vi "TestCloneAPI.vi"() -> ()   [LabVIEW 2014, in "PmuImpairModule.lvlib"]
uses:
  PmuImpairModule.lvlib
  PmuImpairPlugins/PmuImpairPluginBase_class/TypeDefs/clImpairConfig.ctl
  PublicAPI/Arguments/Requests/dblImpairParams.ctl
  EventPlugins/EventPluginBaseClass/TypeDefs/clEvtReportArray.ctl
  EventPlugins/EventPluginBaseClass/TypeDefs/clEvtReport.ctl
  EventPlugins/EventPluginBaseClass/TypeDefs/dblEvtSignalArray.ctl
  EventPlugins/EventPluginBaseClass/TypeDefs/clEvtConfig.ctl
  <userlib>/NIST/ModuleAdminLib/ModuleAdmin/ModuleAdmin.lvclass
  PublicAPI/Arguments/Broadcasts/clDidInit.ctl
  <userlib>/NIST/ModuleAdminLib/ModuleAdmin/ModuleAdmin.lvclass/ModuleAdmin.ctl
  PublicAPI/Arguments/Requests/clStopArgument.ctl
  PublicAPI/Arguments/Broadcasts/clStatUpdate.ctl
  PublicAPI/Arguments/Broadcasts/clErrorRpt.ctl
  <userlib>/NIST/ModuleAdminLib/ModuleAdmin/Accessors/Read CloneRegRef.vi
  <userlib>/NIST/ModuleAdminLib/CloneRegistration/CloneRegistration.lvclass
  PmuImpairPlugins/PmuImpairPluginBase_class/PmuImpairPluginBase.lvclass
  EventPlugins/EventPluginBaseClass/EventPluginBaseClass.lvclass
panel:
  in  "Show Panel":bool=TRUE
  in  "btnWriteEvtParams":bool caption="Write Impair Config"
  in  "dblEvtParams":dbl[][](array[numeric])=[[70.0, 20.0], [60.0, 60.0], [0.0, 0.0], [0.0, 0.0], [0.0, 0.0], [0.0, 0.0], [0.0, 0.0], [0.0, 0.0], [0.0, 0.0], [0.0, 0.0], [0.0, 0.0], [0.0, 0.0], [0.0, 0.0]]
  in  "btnWriteEventConfig":bool caption="Write Impair Config"
  in  "clEvtConfig":T1={"T0(UTC)"=0.0, "F0"=60.0, "Fs"=60, "FSamp"=960, "bPosSeq"=FALSE}
  in  "dblEventSignalArray":T2=[[98.99494936611666, 91.45940754134637, 70.00000000000001, 37.8837270102338, 2.80427866210764e-14, -37.88372701023376, -70.0, -91.45940754134637, -98.99494936611666, -91.45940754134638, -70.00000000000004, -37.88372701023385, -1.8184476598510646e-14, 37.883727010233734, 69.99999999999999, 91.45940754134634, 98.99494936611666, 91.4594075413464, 70.00000000000009, 37.88372701023394, 1.1823263868380915e-13, -37.883727010233635, -69.99999999999991, -91.45940754134627, -98.99494936611666, -91.45940754134637, -70.0000000000001, -37.88372701023387, -4.2430445396524844e-14, 37.88372701023363, 69.99999999999991, 91.45940754134627, 98.99494936611666, 91.45940754134637, 70.0000000000001, 37.883727010233876, 2.3040378516811477e-13, -37.88372701023378, -69.99999999999977, -91.45940754134632, -98.99494936611666, -91.45940754134644, -70.00000000000024, -37.88372701023389, -2.4252676956712185e-13, 37.88372701023344, 69.99999999999964, 91.45940754134625, 98.99494936611666, 91.45940754134644, 70.0, 37.8837270102339, 2.546497539661289e-13, -37.883727010233436, -69.99999999999989, -91.45940754134625, -98.99494936611666, -91.45940754134645, -70.00000000000026, -37.88372701023424, -2.6677273836513605e-13, 37.88372701023342, 69.99999999999962, 91.45940754134624, 98.99494936611666, 91.45940754134658, 70.00000000000001, 37.883727010233926, 2.7889572276414313e-13, -37.883727010233414, -69.99999999999986, -91.45940754134624, -98.99494936611666, -91.4594075413466, -70.00000000000001, -37.88372701023393, -6.427194179083158e-13, 37.88372701023307, 69.99999999999986, 91.45940754134622, 98.99494936611666, 91.45940754134645, 70.00000000000028, 37.88372701023427, 6.548424023073229e-13, -37.88372701023371, -69.99999999999986, -91.45940754134622, -98.99494936611666, -91.45940754134632, -70.00000000000054, -37.88372701023461, -1.0186660974514956e-12, 37.88372701023337, 69.99999999999959, 91.45940754134608, 98.99494936611666, 91.45940754134647, 70.0000000000003, 37.883727010234296, -2.431305038499409e-14, -37.883727010233684, -69.99999999999983, -91.45940754134621, -98.99494936611666, -91.45940754134661, -70.00000000000054, -37.88372701023463, -3.3951064475917863e-13, 37.88372701023335, 69.99999999999957, 91.45940754134607, 98.99494936611666, 91.45940754134648, 70.00000000000031, 37.88372701023432, 7.033343399033513e-13, -37.88372701023302, -69.99999999999932, -91.45940754134621, -98.99494936611666, -91.45940754134661, -70.00000000000057, -37.88372701023465, -1.0671580350475241e-12, 37.88372701023333, 69.99999999999956, 91.45940754134607, 98.99494936611666, 91.45940754134675, 70.00000000000082, 37.88372701023499, 2.41788872110343e-14, -37.88372701023364, -69.9999999999998, -91.4594075413462, -98.99494936611666, -91.45940754134662, -70.0000000000006, -37.88372701023468, -3.8800258235520704e-13, 37.88372701023331, 69.99999999999953, 91.45940754134607, 98.99494936611666, 91.45940754134676, 70.00000000000084, 37.88372701023371, 4.8424856009048493e-14, -37.88372701023362, -69.99999999999977, -91.45940754134593, -98.99494936611666, -91.4594075413469, -70.0000000000011, -37.88372701023405, -4.122485511532212e-13, 37.88372701023329, 69.99999999999952, 91.45940754134605, 98.99494936611666, 91.45940754134678, 70.00000000000036, 37.88372701023439, 7.760722462973939e-13, -37.88372701023295, -69.99999999999926, -91.45940754134591, -98.99494936611666, -91.4594075413469, -70.00000000000011, -37.88372701023407, -4.364945199512354e-13, 37.883727010233265, 69.9999999999995, 91.45940754134604, 98.99494936611666, 91.45940754134625, 69.99999999999989, 37.883727010233756, 1.5037196365857394e-12, -37.88372701023228, -69.99999999999875, -91.45940754134563, -98.99494936611666, -91.45940754134665, -70.00000000000064, -37.88372701023474, -1.1641419102395808e-12, 37.88372701023259, 69.99999999999899, 91.45940754134577, 98.99494936611666], [28.284271247461902, 26.13125929752753, 20.000000000000004, 10.823922002923942, 8.012224748878971e-15, -10.823922002923933, -20.0, -26.13125929752753, -28.284271247461902, -26.13125929752754, -20.00000000000001, -10.823922002923956, -5.1955647424316135e-15, 10.823922002923924, 19.999999999999996, 26.131259297527524, 28.284271247461902, 26.131259297527542, 20.000000000000025, 10.823922002923982, 3.3780753909659755e-14, -10.823922002923897, -19.99999999999998, -26.131259297527503, -28.284271247461902, -26.13125929752753, -20.00000000000003, -10.823922002923963, -1.2122984399007097e-14, 10.823922002923894, 19.999999999999975, 26.131259297527503, 28.284271247461902, 26.13125929752753, 20.000000000000032, 10.823922002923965, 6.582965290517564e-14, -10.823922002923938, -19.999999999999936, -26.13125929752752, -28.284271247461902, -26.131259297527553, -20.000000000000068, -10.823922002923968, -6.929336273346338e-14, 10.823922002923842, 19.999999999999897, 26.1312592975275, 28.284271247461902, 26.131259297527553, 20.0, 10.823922002923972, 7.275707256175113e-14, -10.823922002923839, -19.999999999999968, -26.1312592975275, -28.284271247461902, -26.131259297527556, -20.00000000000007, -10.823922002924068, -7.622078239003887e-14, 10.823922002923835, 19.999999999999893, 26.131259297527496, 28.284271247461902, 26.131259297527595, 20.000000000000004, 10.823922002923979, 7.968449221832661e-14, -10.823922002923831, -19.99999999999996, -26.131259297527496, -28.284271247461902, -26.131259297527595, -20.000000000000004, -10.82392200292398, -1.8363411940237595e-13, 10.823922002923736, 19.999999999999957, 26.131259297527492, 28.284271247461902, 26.13125929752756, 20.00000000000008, 10.823922002924077, 1.870978292306637e-13, -10.823922002923918, -19.999999999999957, -26.131259297527492, -28.284271247461902, -26.13125929752752, -20.000000000000153, -10.823922002924174, -2.9104745641471305e-13, 10.82392200292382, 19.999999999999883, 26.131259297527453, 28.284271247461902, 26.131259297527563, 20.000000000000085, 10.823922002924085, -6.9465858242840266e-15, -10.823922002923911, -19.99999999999995, -26.13125929752749, -28.284271247461902, -26.131259297527603, -20.000000000000156, -10.823922002924181, -9.700304135976532e-14, 10.823922002923815, 19.99999999999988, 26.13125929752745, 28.284271247461902, 26.131259297527567, 20.00000000000009, 10.82392200292409, 2.0095266854381467e-13, -10.82392200292372, -19.999999999999805, -26.131259297527485, -28.284271247461902, -26.131259297527603, -20.000000000000163, -10.823922002924187, -3.04902295727864e-13, 10.823922002923808, 19.999999999999872, 26.13125929752745, 28.284271247461902, 26.131259297527645, 20.000000000000234, 10.823922002924283, 6.908253488866942e-15, -10.823922002923897, -19.999999999999943, -26.131259297527485, -28.284271247461902, -26.131259297527606, -20.000000000000167, -10.823922002924194, -1.108578806729163e-13, 10.823922002923803, 19.99999999999987, 26.131259297527446, 28.284271247461902, 26.13125929752765, 20.00000000000024, 10.823922002923918, 1.3835673145442426e-14, -10.823922002923892, -19.999999999999936, -26.131259297527407, -28.284271247461902, -26.131259297527688, -20.000000000000313, -10.823922002924014, -1.1778530032949179e-13, 10.823922002923796, 19.999999999999865, 26.131259297527443, 28.284271247461902, 26.13125929752765, 20.000000000000103, 10.82392200292411, 2.2173492751354114e-13, -10.8239220029237, -19.999999999999787, -26.131259297527404, -28.284271247461902, -26.131259297527688, -20.000000000000032, -10.82392200292402, -1.2471271998606725e-13, 10.823922002923789, 19.999999999999858, 26.13125929752744, 28.284271247461902, 26.1312592975275, 19.999999999999968, 10.823922002923931, 4.2963418188163984e-13, -10.823922002923508, -19.999999999999645, -26.131259297527325, -28.284271247461902, -26.131259297527617, -20.00000000000018, -10.823922002924212, -3.32611974354166e-13, 10.823922002923599, 19.999999999999712, 26.13125929752736, 28.284271247461902]]
  in  "btnWriteEvtSignal":bool caption="Write Impair Config"
  in  "btnReadPathToPlugin":bool caption="Write Impair Config"
  out "PathToPluginIniFileReport":path=path "P:/Framework/PmuImpairment/PmuImpairPlugins/SineModelPlugin/SineModelPlugin.ini"
  in  "btnGetImpairReports":bool caption="Write Impair Config"
  out "ImpairReportArray":T3 {"Synx" format="%#_4g"}
  in  "btnWriteEvtReports":bool caption="Write Impair Config"
  in  "EvtReportArray":T3=[{"Timestamp"=0.0, "Synx"=[70.0+0.0i, 35.0-60.6218i, 35.0+60.6218i], "Freq"=59.9, "ROCOF"=0.0, "ID"=0}, {"Timestamp"=0.02, "Synx"=[69.9962-0.733i, 34.3633-60.985i, 35.6329+60.2519i], "Freq"=59.9, "ROCOF"=0.0, "ID"=0}, {"Timestamp"=0.03, "Synx"=[69.9846-1.466i, 33.7228-61.3415i, 36.2619+59.8755i], "Freq"=59.9, "ROCOF"=0.0, "ID"=0}, {"Timestamp"=0.05, "Synx"=[69.9655-2.1988i, 33.0786-61.6912i, 36.8869+59.4925i], "Freq"=59.9, "ROCOF"=0.0, "ID"=0}] {"Synx" format="%#_4g"}
  in  "btnReadImpairParams":bool caption="Write Impair Config"
  out "dblImpairParamsReport":T5
  in  "btnWriteImpairParams":bool caption="Write Impair Config"
  in  "dblImpairParams":T5=[[8.19], [164.0]]
  in  "btnReadImpairConfig":bool caption="Write Impair Config"
  out "clImpairConfigReport":T6={"FilterType"="", "bPosSeq"=TRUE}
  in  "btnWriteImpairConfig":bool caption="Write Impair Config"
  in  "btnLoadPlugin":bool
  in  "PathToPluginIniFile":path=path "D:/Projects/PARTF/Framework/PmuImpairment/PmuImpairPlugins/C37BehaviourPlugin/C37BehaviourPlugin.ini"
  in  "clImpairConfig":T6={"FilterType"="Hamming", "bPosSeq"=TRUE}
  in  "btnRemove":bool
  out "Status Log":string
  out "Active Modules (Array)":string[](array[string])
  in  "btnAdd":bool
  in  "btnStop":bool
  in  "Select Module":i32(ring)=-1 caption="Select Module to send Request" items=["All"=-1]
  # "Hidden"
  # "Visible"
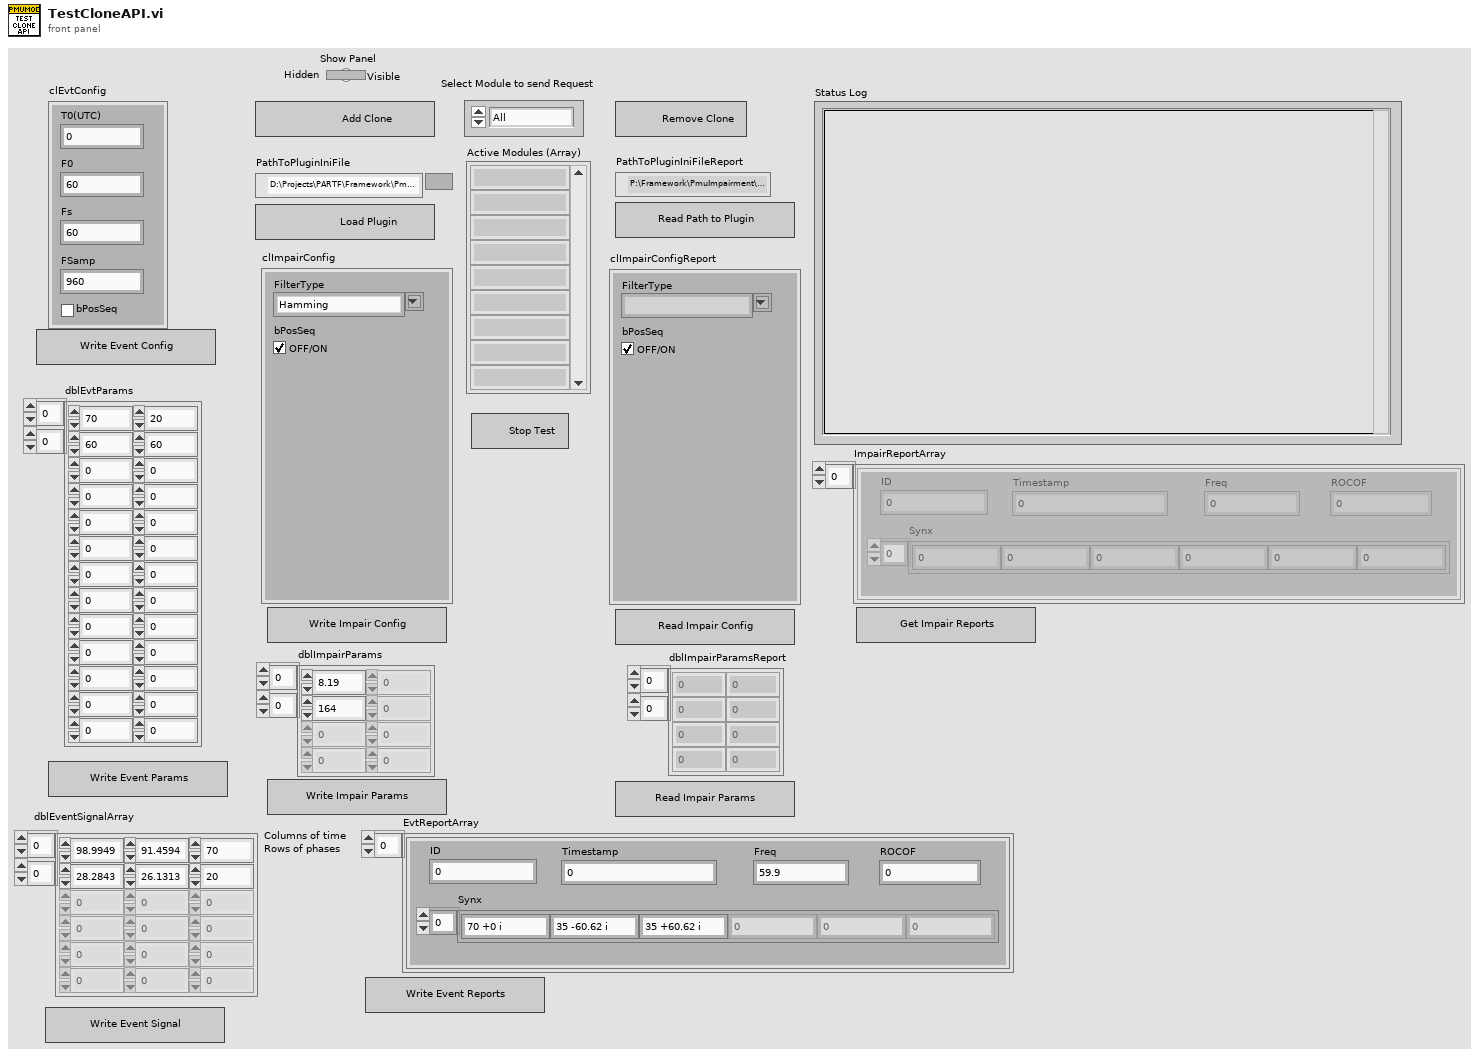
[diagram p1: front panel]
types:
  T1 = typedef "EventPlugins.lvlib/EventPluginBaseClass.lvclass/clEvtConfig.ctl" = cluster{"T0(UTC)":dbl, "F0":dbl, "Fs":i32, "FSamp":u32, "bPosSeq":bool}
  T2 = typedef "EventPlugins.lvlib/EventPluginBaseClass.lvclass/dblEvtSignalArray.ctl" = dbl[][]
  T3 = typedef "EventPlugins.lvlib/EventPluginBaseClass.lvclass/clEvtReportArray.ctl" = T4[]
  T4 = typedef "EventPlugins.lvlib/EventPluginBaseClass.lvclass/clEvtReport.ctl" = cluster{"Timestamp":dbl, "Synx":cdb[], "Freq":dbl, "ROCOF":dbl, "ID":i16}
  T5 = typedef "PmuImpairModule.lvlib/dblImpairParams.ctl" = dbl[][]
  T6 = typedef "PmuImpairPlugins.lvlib/PmuImpairPluginBase.lvclass/clImpairConfig.ctl" = cluster{"FilterType":string, "bPosSeq":bool}
  T7 = typedef "PmuImpairModule.lvlib/clBroadcastEvents.ctl" = cluster{"DidInit":refnum<user-event>, "StatusUpdate":refnum<user-event>, "ErrorReport":refnum<user-event>, "DidStop":refnum<user-event>, "ImpairConfig":refnum<user-event>, "ImpairParams":refnum<user-event>, "ImpairReports":refnum<user-event>, "PathToPlugin":refnum<user-event>, "BusNumber":refnum<user-event>}
  T8 = typedef "PmuImpairModule.lvlib/clDidInit.ctl" = cluster{"Init?":bool, "ModuleAdmin":refnum<class "ModuleAdmin.lvclass">}
  T9 = typedef "PmuImpairModule.lvlib/clStopArgument.ctl" = cluster{"Exit via Stop Module Req?":bool, "Wait for Module to stop?":bool, "ModuleAdmin":refnum<class "ModuleAdmin.lvclass">}
  T10 = typedef "PmuImpairModule.lvlib/clStatUpdate.ctl" = cluster{"Status":string}
  T11 = typedef "PmuImpairModule.lvlib/clErrorRpt.ctl" = cluster{"error":errorcluster, "AdditionalInfo":string}
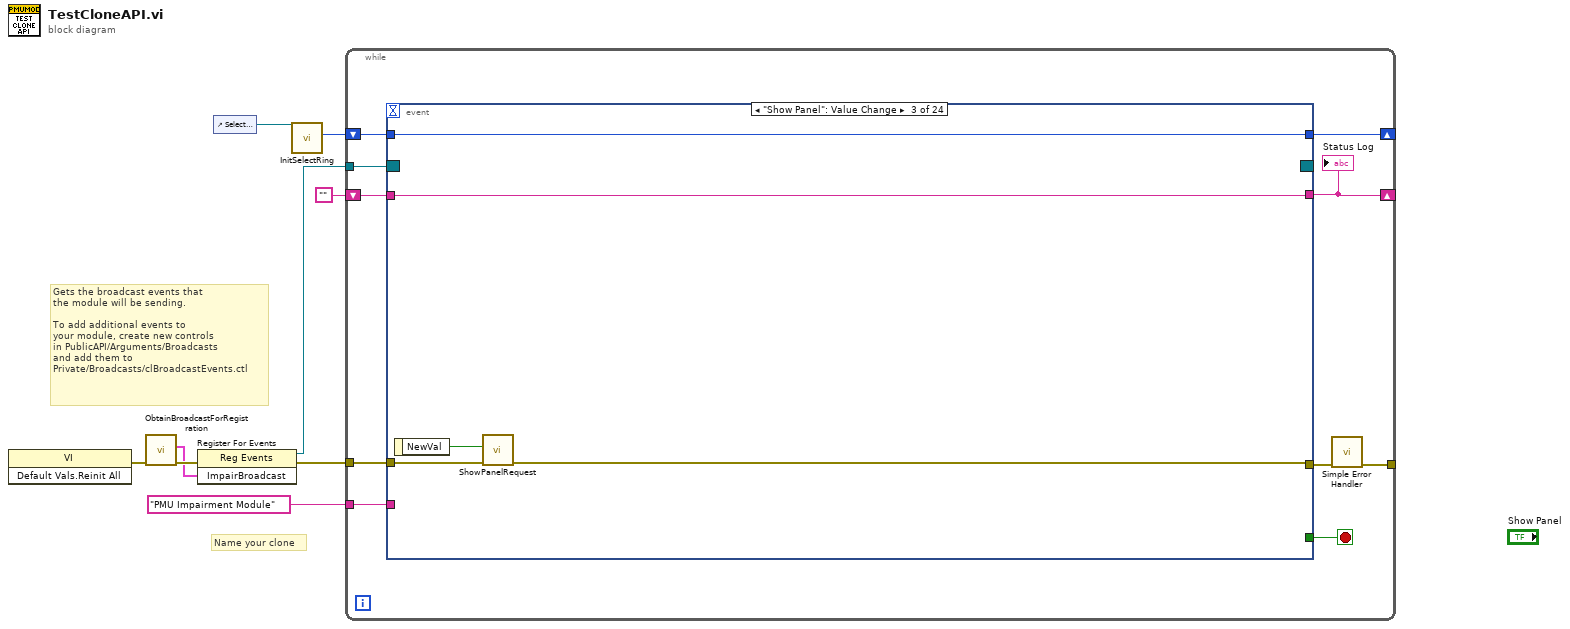
[diagram p0: block diagram]
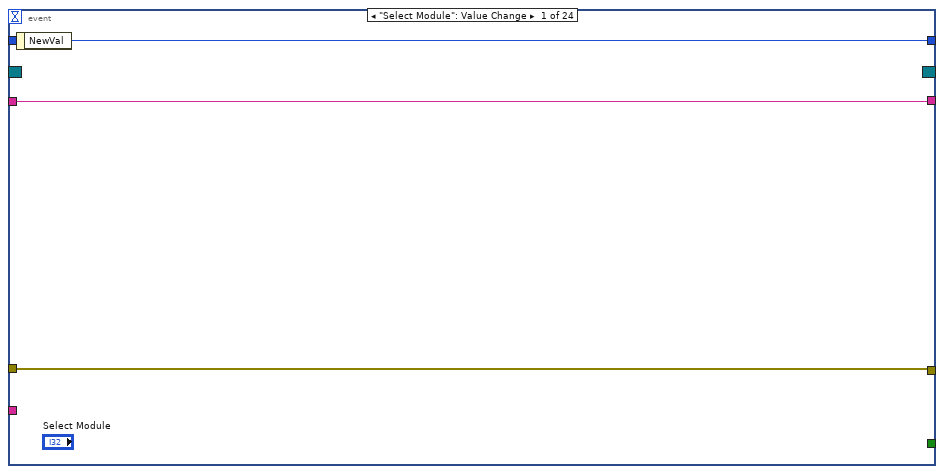
[diagram p2: hidden frame]
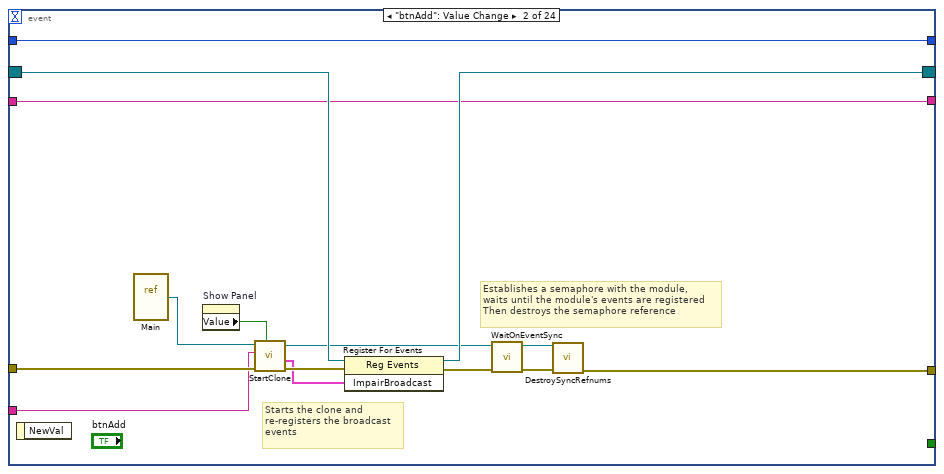
[diagram p3: hidden frame]
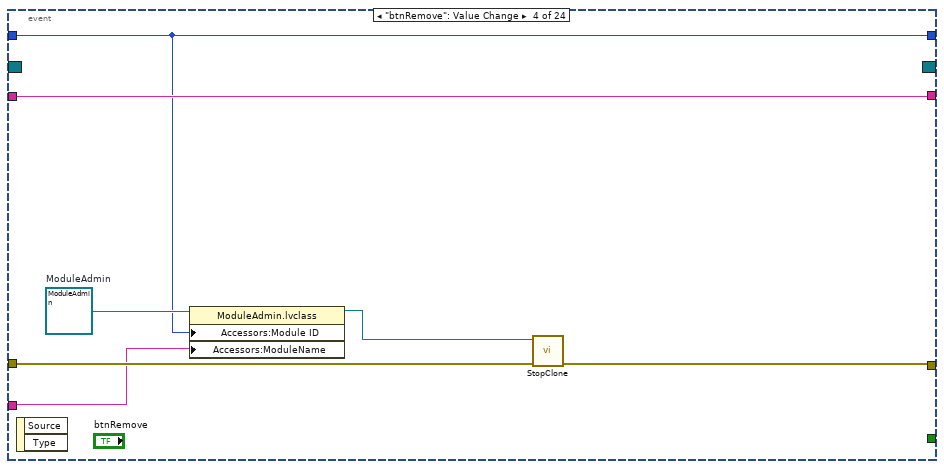
[diagram p4: hidden frame]
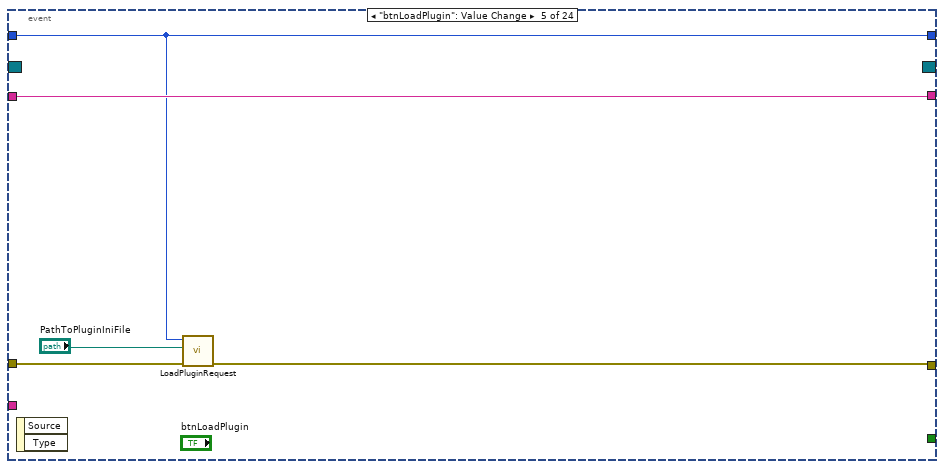
[diagram p5: hidden frame]
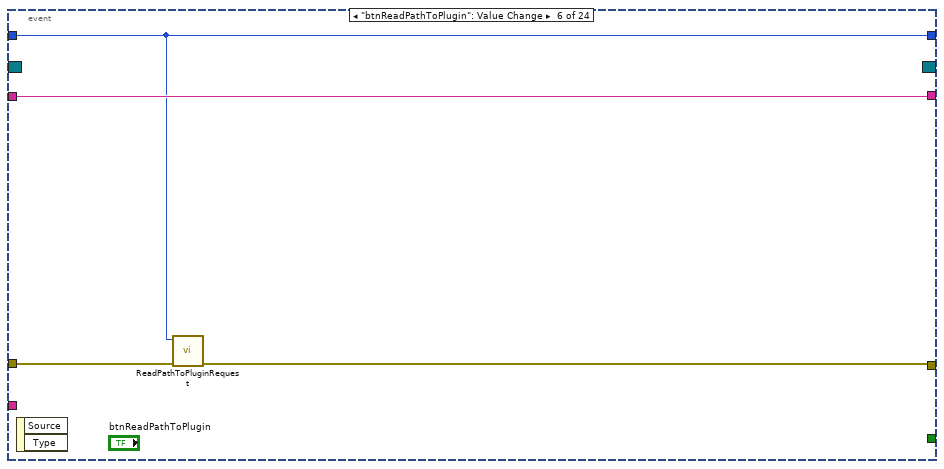
[diagram p6: hidden frame]
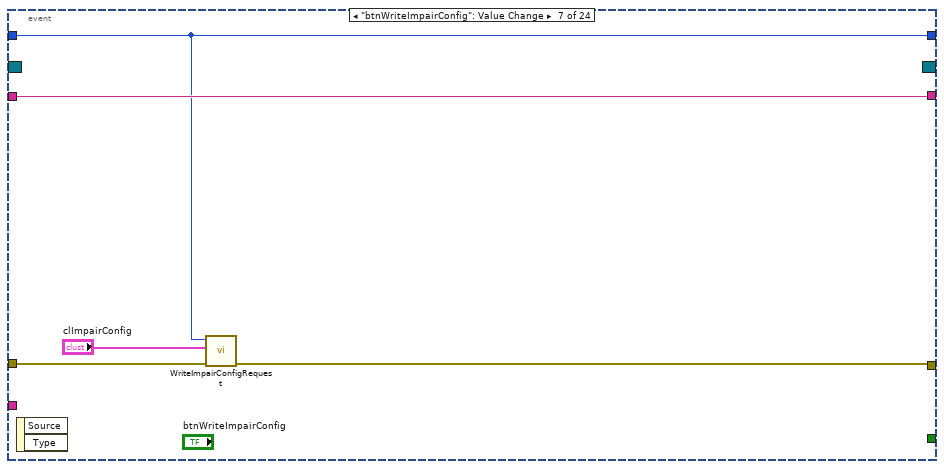
[diagram p7: hidden frame]
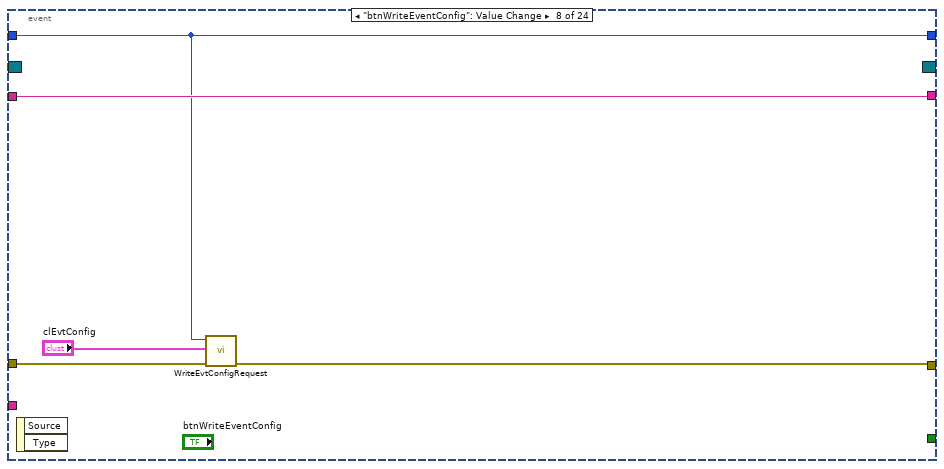
[diagram p8: hidden frame]
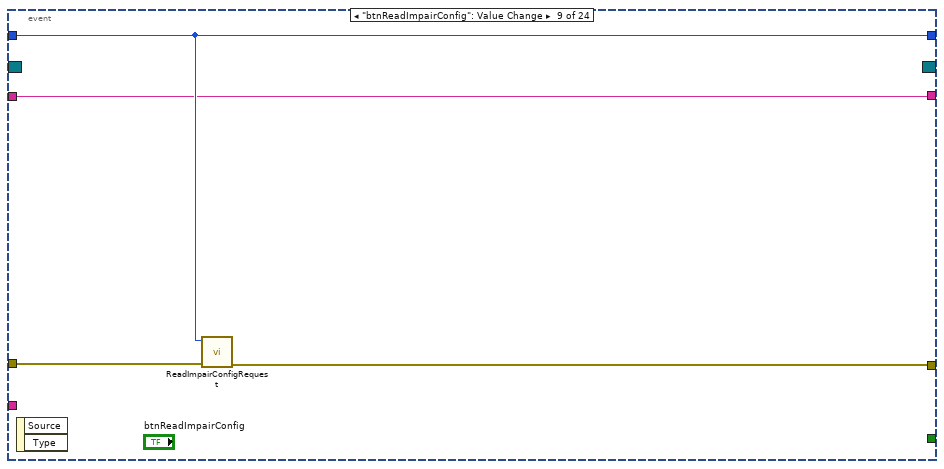
[diagram p9: hidden frame]
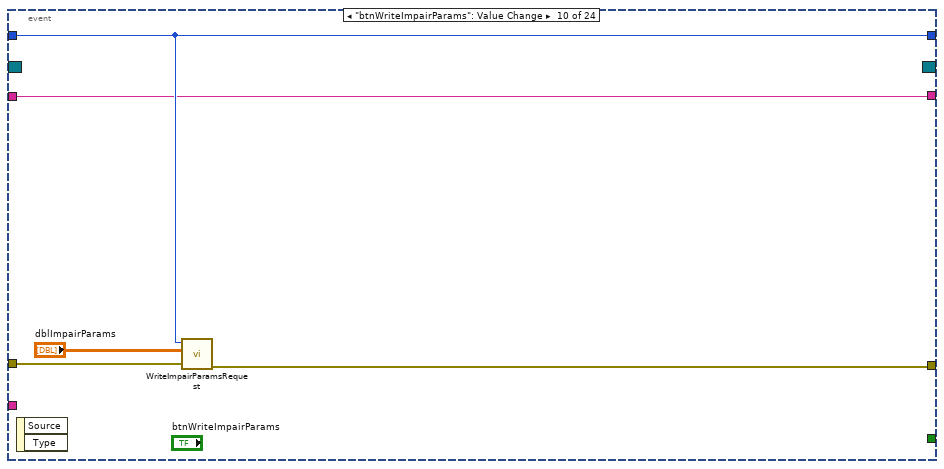
[diagram p10: hidden frame]
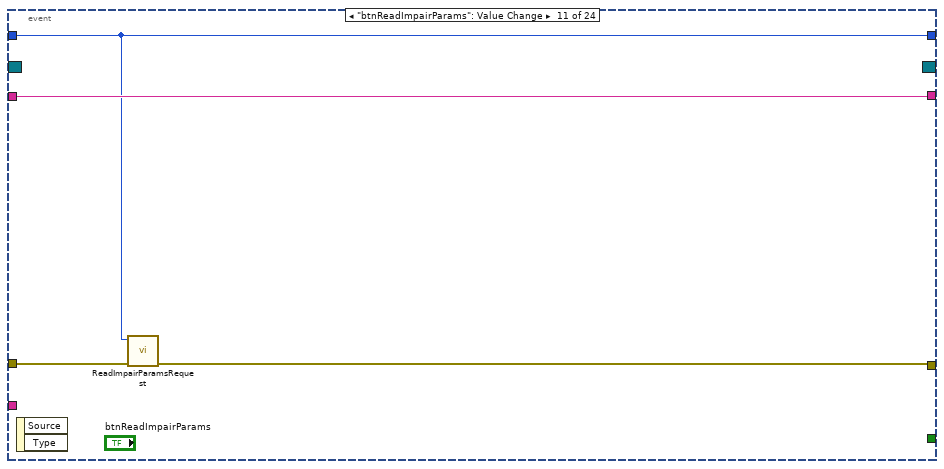
[diagram p11: hidden frame]
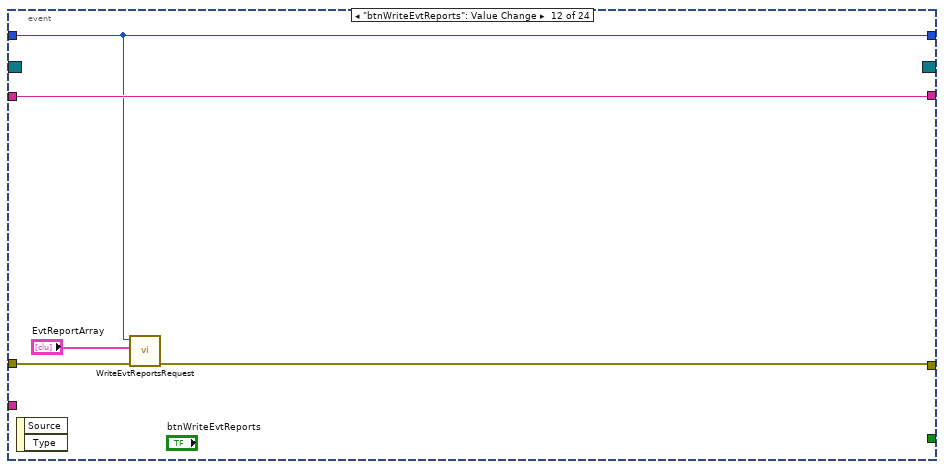
[diagram p12: hidden frame]
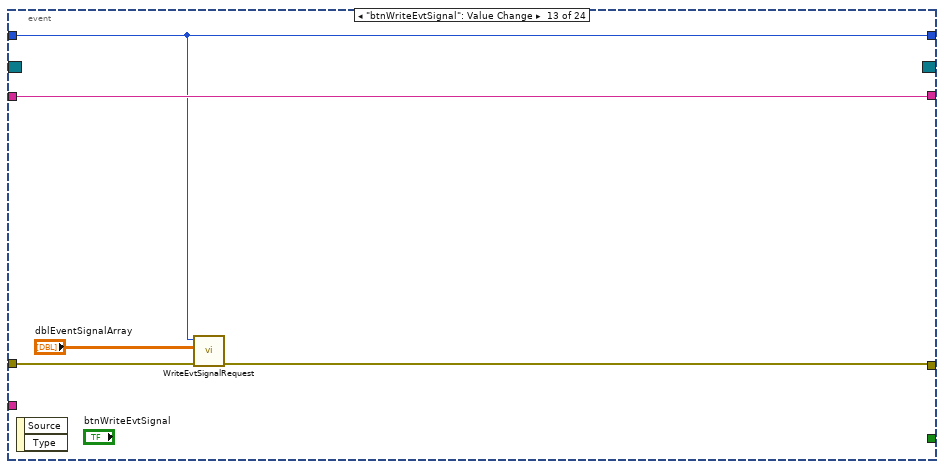
[diagram p13: hidden frame]
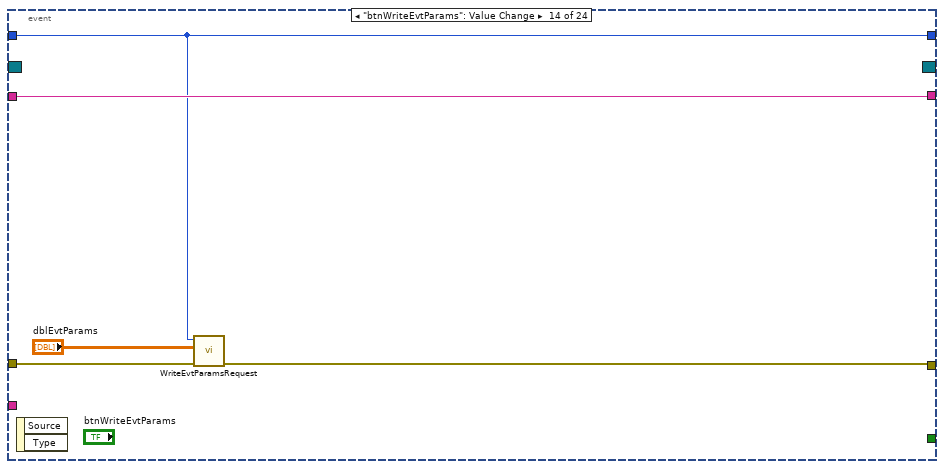
[diagram p14: hidden frame]
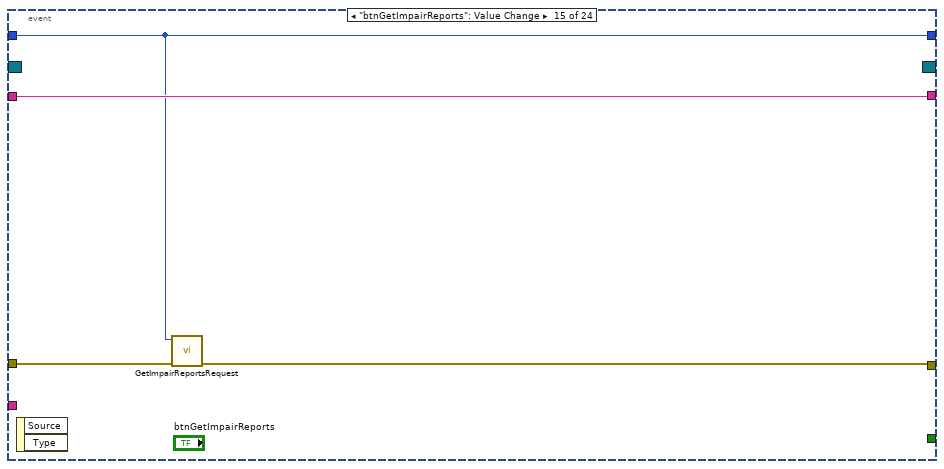
[diagram p15: hidden frame]
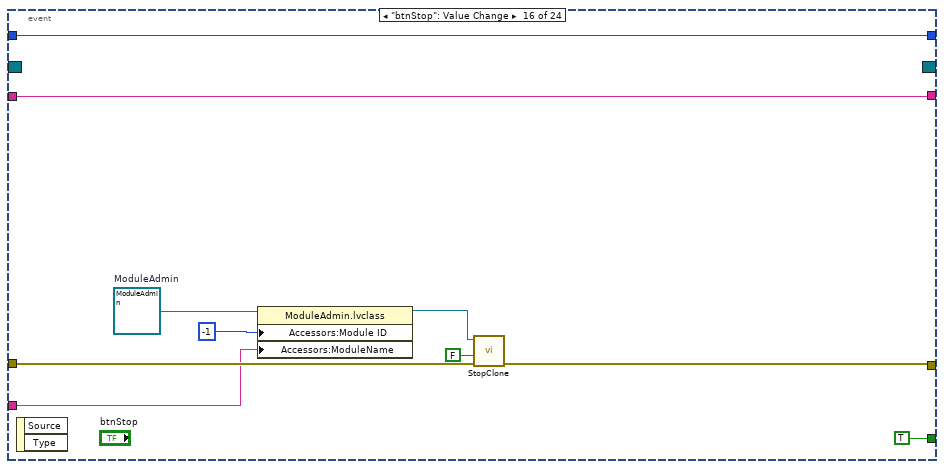
[diagram p16: hidden frame]
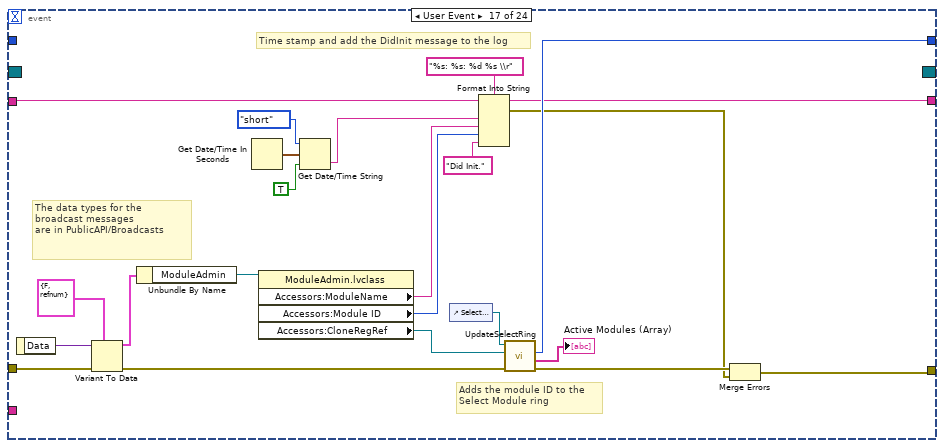
[diagram p17: hidden frame]
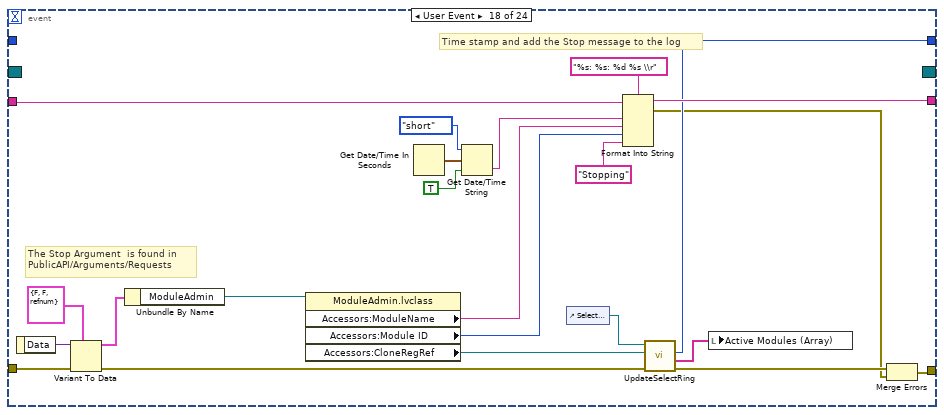
[diagram p18: hidden frame]
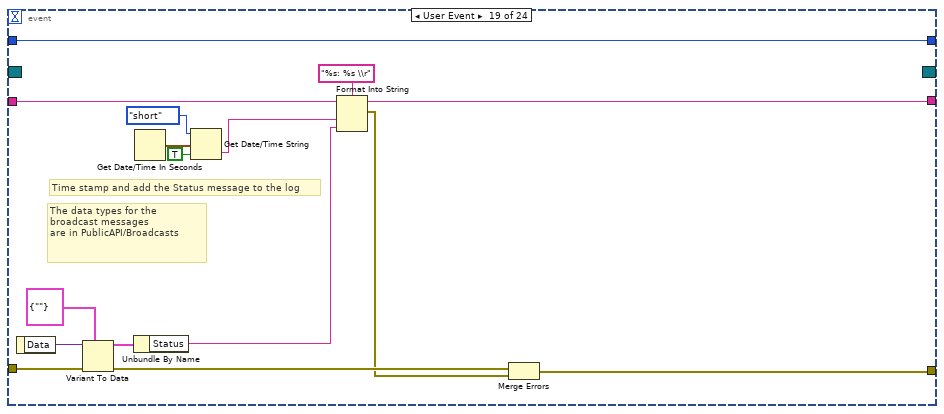
[diagram p19: hidden frame]
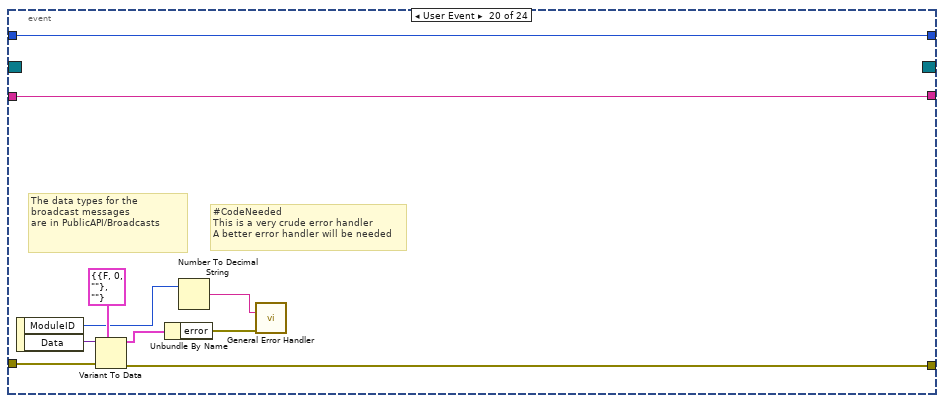
[diagram p20: hidden frame]
diagram:
  # "Name your clone"
  # "Gets the broadcast events that\nthe module will be sending.\n\nTo add additional events to\nyour module, create new controls\nin PublicAPI/Arguments/Broadcasts\nand add them to\nPrivate/Broadcasts/clBroadcastEvents.ctl"
  n1 = invoke class="VI" method="Default Vals.Reinit All"() -> (error out=w7:errorcluster)  [unwired: 3 in, 2 out]
  n2 = call "ObtainBroadcastForRegistration.vi"("error in (no error)"=w7) -> ("error out"=w6:errorcluster, "ImpairBroadcast"=w5:T7)  [unwired: 9 in]
  n3 = register-events(error in=w6, w5) -> (reference out=w3:refnum<event-registration>, error out=w4:errorcluster)  [unwired: 1 in]
  n4 = control-ref of="Select Module"() -> (w9:refnum<vi>)
  n5 = call "InitSelectRing.vi"("Ring Refnum"=w9) -> ("Module Ring Value"=w8:i32)  [unwired: 9 in, 1 out]
  n6 = while {
    shift-right: [w18] -> _
    shift-left: w8 -> [w19]
    tunnel: w4 -> [w16]
    tunnel: w3 -> [w13]
    tunnel: [w14] -> _
    shift-right: [w12] -> _
    shift-left: "" -> [w11]
    tunnel: "PMU Impairment Module" ("ModuleName") -> [w10]
    stop <- w17 stop-if-true
    n7 = event shown="[2] \"Show Panel\": Value Change" {
      selector: w13 -> [_ w29 _ _ _ _ _ _ _ _ _ _ _ _ _ _ _ _ _ _ _ _ _ _]
      dyn-events: [_ w28 _ _ _ _ _ _ _ _ _ _ _ _ _ _ _ _ _ _ _ _ _ _] -> _
      timeout: _ -> [_ _ _ _ _ _ _ _ _ _ _ _ _ _ _ _ _ _ _ _ _ _ _ _]
      tunnel: w19 -> [_ w37 w38 w44 w51 w55 w60 w66 w71 w74 w78 w83 w89 w94 w98 w110 _ _ w172 w174 w184 w190 w197 w204]
      tunnel: [w22 w37 w38 w44 w51 w55 w60 w66 w71 w74 w78 w83 w89 w94 w98 w110 w128 w143 w172 w174 w184 w190 w197 w204] -> w18
      tunnel: [_ _ _ _ _ _ _ _ _ _ _ _ _ _ _ TRUE _ _ _ _ _ _ _ _] -> w17
      tunnel: w16 -> [w20 w36 w41 w48 w53 w58 w63 w68 w72 w77 w81 w85 w90 w95 w100 w108 w133 w152 w169 w181 w189 w196 w203 w210]
      tunnel: [w20 w30 w40 w47 w50 w57 w59 w65 w69 w76 w80 w82 w88 w93 w97 w106 w117 w140 w160 w180 w186 w193 w202 w209] -> w15
      tunnel: [w21 w26 w39 w49 w54 w56 w61 w67 w70 w73 w79 w86 w91 w96 w99 w105 w121 w149 w163 w173 w185 w191 w198 w205] -> w12
      tunnel: w11 -> [w21 w26 w39 w49 w54 w56 w61 w67 w70 w73 w79 w86 w91 w96 w99 w105 w120 w150 w171 w173 w185 w191 w198 w205]
      tunnel: w10 -> [_ w25 _ w45 _ _ _ _ _ _ _ _ _ _ _ w102 _ _ _ _ _ _ _ _]
      event "Select Module": Value Change {
        n8 = event-data() -> ("NewVal"=w22:i32)  [unwired: 1 in]
      }
      event "btnAdd": Value Change {
        # "Establishes a semaphore with the module,\nwaits until the module's events are registered\nThen destroys the semaphore reference"
        # "Starts the clone and\nre-registers the broadcast \nevents"
        n9 = event-data() -> ()  [unwired: 1 in, 1 out]
        n10 = vi-ref "Main.vi"() -> (w27:refnum<vi>)
        n11 = property on="Show Panel" class="Bool (strict)"() -> ("Value"=w23:bool)  [unwired: 2 in, 2 out]
        n12 = call "StartClone.vi"("ShowPanel? (f)"=w23, "error in (no error)"=w36, "ModuleName"=w25, "VI Refnum"=w27) -> ("error out"=w35:errorcluster, "clBroadcastEvents"=w31:T7, "ModuleAdmin"=w24:refnum<class "ModuleAdmin.lvclass">)  [unwired: 5 in]
        n13 = register-events(reference=w29, error in=w35, w31) -> (reference out=w28:refnum<event-registration>, error out=w34:errorcluster)
        n14 = call <userlib>:"WaitOnEventSync.vi"("error in (no error)"=w34, "ModuleAdmin"=w24) -> ("error out"=w33:errorcluster, "ModuleAdmin"=w32:refnum<class "ModuleAdmin.lvclass">)  [unwired: 8 in]
        n15 = call <userlib>:"DestroySyncRefnums.vi"("error in (no error)"=w33, "ModuleAdmin"=w32) -> ("error out"=w30:errorcluster)  [unwired: 9 in]
      }
      event "Show Panel": Value Change {
        n16 = event-data() -> ("NewVal"=w42:bool)  [unwired: 1 in]
        n17 = call "ShowPanelRequest.vi"("error in (no error)"=w41, "ShowPanel?"=w42) -> ("error out"=w40:errorcluster)  [unwired: 9 in]
      }
      event "btnRemove": Value Change {
        w46 = refnum<class "ModuleAdmin.lvclass"> refnum  # ModuleAdmin
        n18 = event-data() -> ()  [unwired: 1 in, 2 out]
        n19 = property class="ModuleAdmin.lvclass"(reference=w46, "Accessors:Module ID"=w44, "Accessors:ModuleName"=w45) -> (reference out=w43:refnum<class "ModuleAdmin.lvclass">)  [unwired: 1 in, 1 out]
        n20 = call "StopClone.vi"("error in (no error)"=w48, "ModuleAdmin"=w43) -> ("error out"=w47:errorcluster)  [unwired: 9 in]
      }
      event "btnLoadPlugin": Value Change {
        n21 = event-data() -> ()  [unwired: 1 in, 2 out]
        n22 = call "LoadPluginRequest.vi"("error in (no error)"=w53, "PathToPlugin"="PathToPluginIniFile", "ModuleID"=w51) -> ("error out"=w50:errorcluster)  [unwired: 8 in]
      }
      event "btnReadPathToPlugin": Value Change {
        n23 = event-data() -> ()  [unwired: 1 in, 2 out]
        n24 = call "ReadPathToPluginRequest.vi"("error in (no error)"=w58, "ModuleID"=w55) -> ("error out"=w57:errorcluster)  [unwired: 9 in]
      }
      event "btnWriteImpairConfig": Value Change {
        n25 = event-data() -> ()  [unwired: 1 in, 2 out]
        n26 = call "WriteImpairConfigRequest.vi"("error in (no error)"=w63, "clImpairConfig"="clImpairConfig", "ModuleID"=w60) -> ("error out"=w59:errorcluster)  [unwired: 8 in]
      }
      event "btnWriteEventConfig": Value Change {
        n27 = event-data() -> ()  [unwired: 1 in, 2 out]
        n28 = call "WriteEvtConfigRequest.vi"("error in (no error)"=w68, "EvtConfig"="clEvtConfig", "ModuleID"=w66) -> ("error out"=w65:errorcluster)  [unwired: 8 in]
      }
      event "btnReadImpairConfig": Value Change {
        n29 = event-data() -> ()  [unwired: 1 in, 2 out]
        n30 = call "ReadImpairConfigRequest.vi"("error in (no error)"=w72, "ModuleID"=w71) -> ("error out"=w69:errorcluster)  [unwired: 9 in]
      }
      event "btnWriteImpairParams": Value Change {
        n31 = event-data() -> ()  [unwired: 1 in, 2 out]
        n32 = call "WriteImpairParamsRequest.vi"("error in (no error)"=w77, "dblImpairParams"="dblImpairParams", "ModuleID"=w74) -> ("error out"=w76:errorcluster)  [unwired: 8 in]
      }
      event "btnReadImpairParams": Value Change {
        n33 = event-data() -> ()  [unwired: 1 in, 2 out]
        n34 = call "ReadImpairParamsRequest.vi"("error in (no error)"=w81, "ModuleID"=w78) -> ("error out"=w80:errorcluster)  [unwired: 9 in]
      }
      event "btnWriteEvtReports": Value Change {
        n35 = event-data() -> ()  [unwired: 1 in, 2 out]
        n36 = call "WriteEvtReportsRequest.vi"("error in (no error)"=w85, "EvtReportArray"="EvtReportArray", "ModuleID"=w83) -> ("error out"=w82:errorcluster)  [unwired: 8 in]
      }
      event "btnWriteEvtSignal": Value Change {
        n37 = event-data() -> ()  [unwired: 1 in, 2 out]
        n38 = call "WriteEvtSignalRequest.vi"("error in (no error)"=w90, "EvtSignalArray"="dblEventSignalArray", "ModuleID"=w89) -> ("error out"=w88:errorcluster)  [unwired: 8 in]
      }
      event "btnWriteEvtParams": Value Change {
        n39 = event-data() -> ()  [unwired: 1 in, 2 out]
        n40 = call "WriteEvtParamsRequest.vi"("error in (no error)"=w95, "EvtParams"="dblEvtParams", "ModuleID"=w94) -> ("error out"=w93:errorcluster)  [unwired: 8 in]
      }
      event "btnGetImpairReports": Value Change {
        n41 = event-data() -> ()  [unwired: 1 in, 2 out]
        n42 = call "GetImpairReportsRequest.vi"("error in (no error)"=w100, "ModuleID"=w98) -> ("error out"=w97:errorcluster)  [unwired: 9 in]
      }
      event "btnStop": Value Change {
        w104 = refnum<class "ModuleAdmin.lvclass"> refnum  # ModuleAdmin
        n43 = event-data() -> ()  [unwired: 1 in, 2 out]
        n44 = property class="ModuleAdmin.lvclass"(reference=w104, "Accessors:Module ID"=-1 ("Module ID"), "Accessors:ModuleName"=w102) -> (reference out=w101:refnum<class "ModuleAdmin.lvclass">)  [unwired: 1 in, 1 out]
        n45 = call "StopClone.vi"("error in (no error)"=w108, "Wait for Module to stop?"=FALSE, "ModuleAdmin"=w101) -> ("error out"=w106:errorcluster)  [unwired: 8 in]
      }
      event User Event {
        # "Adds the module ID to the \nSelect Module ring"
        # "Time stamp and add the DidInit message to the log"
        # "The data types for the broadcast messages\nare in PublicAPI/Broadcasts"
        n46 = event-data() -> ("Data"=w132:variant)  [unwired: 1 in]
        n47 = Variant To Data(error in=w133, type=T8 {"Init?"=FALSE, "ModuleAdmin"=refnum} ("clDidInit"), Variant=w132) -> (data=w125:T8, error out=w130:errorcluster)
        n48 = Unbundle By Name(w125) -> ("ModuleAdmin"=w114:refnum<class "ModuleAdmin.lvclass">)
        n49 = Get Date/Time In Seconds() -> (seconds since 1Jan1904=w123:timestamp)
        n50 = property class="ModuleAdmin.lvclass"(reference=w114) -> ("Accessors:ModuleName"=w113:string, "Accessors:Module ID"=w112:i32, "Accessors:CloneRegRef"=w111:refnum<data-value>)  [unwired: 1 in, 2 out]
        n51 = Get Date/Time String(date format (0)=enum16{"short", "long", "abbreviated"}."short", seconds (now)=w123, want seconds? (F)=TRUE) -> (time string=w126:string)  [unwired: 1 out]
        n52 = control-ref of="Select Module"() -> (w129:refnum<vi>)
        n53 = Format Into String(format string="%s: %s: %d %s \\r", initial string=w120, w126, w113, w112, "Did Init.") -> (resulting string=w121:string, error out=w118:errorcluster)  [unwired: 1 in]
        n54 = call "UpdateSelectRing.vi"("error in (no error)"=w130, "CloneRegRef"=w111, "Ring Refnum"=w129) -> ("error out"=w119:errorcluster, "ActiveModules"=→"Active Modules (Array)":string[], "Module Ring Value"=w128:i32)  [unwired: 6 in]
        n55 = Merge Errors(w119, w118) -> (w117:errorcluster)
      }
      event User Event {
        # "Time stamp and add the Stop message to the log"
        # "The Stop Argument  is found in\nPublicAPI/Arguments/Requests"
        n56 = event-data() -> ("Data"=w151:variant)  [unwired: 1 in]
        n57 = Variant To Data(error in=w152, type=T9 {"Exit via Stop Module Req?"=FALSE, "Wait for Module to stop?"=FALSE, "ModuleAdmin"=refnum} ("Stop Argument"), Variant=w151) -> (data=w147:T9, error out=w146:errorcluster)
        n58 = Unbundle By Name(w147) -> ("ModuleAdmin"=w137:refnum<class "ModuleAdmin.lvclass">)
        n59 = property class="ModuleAdmin.lvclass"(reference=w137) -> ("Accessors:ModuleName"=w134:string, "Accessors:Module ID"=w135:i32, "Accessors:CloneRegRef"=w136:refnum<data-value>)  [unwired: 1 in, 2 out]
        n60 = Get Date/Time In Seconds() -> (seconds since 1Jan1904=w154:timestamp)
        n61 = Get Date/Time String(date format (0)=enum16{"short", "long", "abbreviated"}."short", seconds (now)=w154, want seconds? (F)=TRUE) -> (time string=w156:string)  [unwired: 1 out]
        n62 = control-ref of="Select Module"() -> (w145:refnum<vi>)
        n63 = Format Into String(format string="%s: %s: %d %s \\r", initial string=w150, w156, w134, w135, "Stopping") -> (resulting string=w149:string, error out=w141:errorcluster)  [unwired: 1 in]
        n64 = call "UpdateSelectRing.vi"("error in (no error)"=w146, "CloneRegRef"=w136, "Ring Refnum"=w145) -> ("error out"=w142:errorcluster, "ActiveModules"=w144:string[], "Module Ring Value"=w143:i32)  [unwired: 6 in]
        n65 = local write "Active Modules (Array)"(w144) -> ()
        n66 = Merge Errors(w142, w141) -> (w140:errorcluster)
      }
      event User Event {
        # "Time stamp and add the Status message to the log"
        # "The data types for the broadcast messages\nare in PublicAPI/Broadcasts"
        n67 = event-data() -> ("Data"=w168:variant)  [unwired: 1 in]
        n68 = Variant To Data(error in=w169, type=T10 {"Status"=""} ("clStatUpdate"), Variant=w168) -> (data=w166:T10, error out=w162:errorcluster)
        n69 = Unbundle By Name(w166) -> ("Status"=w164:string)
        n70 = Get Date/Time In Seconds() -> (seconds since 1Jan1904=w165:timestamp)
        n71 = Get Date/Time String(date format (0)=enum16{"short", "long", "abbreviated"}."short", seconds (now)=w165, want seconds? (F)=TRUE) -> (time string=w157:string)  [unwired: 1 out]
        n72 = Format Into String(format string="%s: %s \\r", initial string=w171, w157, w164) -> (resulting string=w163:string, error out=w161:errorcluster)  [unwired: 1 in]
        n73 = Merge Errors(w162, w161) -> (w160:errorcluster)
      }
      event User Event {
        # "#CodeNeeded\nThis is a very crude error handler\nA better error handler will be needed"
        # "The data types for the broadcast messages\nare in PublicAPI/Broadcasts"
        n74 = event-data() -> ("ModuleID"=w177:i32, "Data"=w182:variant)  [unwired: 1 in]
        n75 = Variant To Data(error in=w181, type=T11 {"error"={"status"=FALSE, "code"=0, "source"=""}, "AdditionalInfo"=""} ("Cluster"), Variant=w182) -> (data=w178:T11, error out=w180:errorcluster)
        n76 = Unbundle By Name(w178) -> ("error"=w176:errorcluster)
        n77 = Number To Decimal String(number=w177) -> (decimal integer string=w175:string)  [unwired: 1 in]
        n78 = call <vilib>:"General Error Handler.vi"("[error source] (\" \")"=w175, "error in (no error)"=w176) -> ()  [unwired: 9 in, 5 out]
      }
      event User Event {
        n79 = event-data() -> ("Data"=w188:variant)  [unwired: 1 in]
        n80 = Variant To Data(error in=w189, type=path "", Variant=w188) -> (data=→"PathToPluginIniFileReport":path, error out=w186:errorcluster)
      }
      event User Event {
        n81 = event-data() -> ("Data"=w195:variant)  [unwired: 1 in]
        n82 = Variant To Data(error in=w196, type=T6 {"FilterType"="", "bPosSeq"=TRUE} ("clImpairConfig"), Variant=w195) -> (data=→"clImpairConfigReport":T6, error out=w193:errorcluster)
      }
      event User Event {
        w200 = T5 []  # dblImpairParams
        n83 = event-data() -> ("Data"=w201:variant)  [unwired: 1 in]
        n84 = Variant To Data(error in=w203, type=w200, Variant=w201) -> (data=→"dblImpairParamsReport":T5, error out=w202:errorcluster)
      }
      event User Event {
        w207 = T3 []  # ImpairReportArray
        n85 = event-data() -> ("Data"=w208:variant)  [unwired: 1 in]
        n86 = Variant To Data(error in=w210, type=w207, Variant=w208) -> (data=→"ImpairReportArray":T3, error out=w209:errorcluster)
      }
    }
    "Status Log" <- w12
    n87 = call <vilib>:"Simple Error Handler.vi"("error in (no error)"=w15) -> ("error out"=w14:errorcluster)  [unwired: 4 in, 4 out]
  }
